vi "Deserialized data to complex.vi"(8 "error in (no error)":errorcluster, 11 "Deserialized Data In":refnum<class "3D Array s16.lvclass">) -> (0 "error out":errorcluster, 3 "Complex Data Out":refnum<class "2D Array c32.lvclass">)   [LabVIEW 2020, in "GPU FFT Calculator.lvlib" / "GPU FFT Calculator.lvclass"]
uses:
  GPU FFT Calculator.lvclass
  <vilib>/Natan Biesmans/G2CPU GPU and CPU HPC Toolkit/G2CPU Libraries/Arrays/2DArray/c32/2D Array c32.lvclass
  C:/Program Files/National Instruments/LabVIEW 2026/vi.lib/Natan Biesmans/G2CPU GPU and CPU HPC Toolkit/G2CPU Libraries/Arrays/Array/Array Prototype.lvclass
  <vilib>/Natan Biesmans/G2CPU GPU and CPU HPC Toolkit/G2CPU Libraries/Arrays/3DArray/s16/3D Array s16.lvclass
  <vilib>/Natan Biesmans/G2CPU GPU and CPU HPC Toolkit/G2CPU Libraries/Arrays/Array/Array Prototype.lvclass/Array Prototype.ctl
  c2dea994-931f-4d55-9a20-c830c6c0dc8e.vi
  b42d50d8-b553-4447-b6c3-f1e712b09a3a.vi
  a356b423-7bdc-4f21-90e1-9c0ca5a82237.vi
  d3968e77-9a7a-4b56-abf9-f7dead729653.vi
  <vilib>/Natan Biesmans/G2CPU GPU and CPU HPC Toolkit/G2CPU Libraries/Arrays/Array/G2CPU Get Array Pointer.vi
  c2dea994-931f-4d55-9a20-c830c6c0dc8e.vi/e7247370-a01f-465a-ac0e-4dfefcb1bb87.vi
  c2dea994-931f-4d55-9a20-c830c6c0dc8e.vi/345e91f0-9a5e-4de4-af9c-133346717e4a.vi
  b42d50d8-b553-4447-b6c3-f1e712b09a3a.vi/2e03f477-51b7-4ba0-bb4f-4f838f6557e6.vi
  b42d50d8-b553-4447-b6c3-f1e712b09a3a.vi/0be70a8c-200c-453e-b8ff-fd186066a0ad.vi
  b42d50d8-b553-4447-b6c3-f1e712b09a3a.vi/e82a863a-43d4-4d21-a8d3-9b1c3ad7b341.vi
  b42d50d8-b553-4447-b6c3-f1e712b09a3a.vi/99530adb-fade-452a-867c-88e355f5b47e.vi
  <vilib>/Natan Biesmans/G2CPU GPU and CPU HPC Toolkit/ArrayFire Driver/VIs/release array.vi
  b42d50d8-b553-4447-b6c3-f1e712b09a3a.vi/9eb95f43-766d-4b65-bcfe-7bdf0b763efe.vi
  b42d50d8-b553-4447-b6c3-f1e712b09a3a.vi/125d45d4-836b-469d-8a4a-6adb452f866d.vi
  b42d50d8-b553-4447-b6c3-f1e712b09a3a.vi/8038e9ed-2e71-4568-91ba-0d873494c5ed.vi
  a356b423-7bdc-4f21-90e1-9c0ca5a82237.vi/2e03f477-51b7-4ba0-bb4f-4f838f6557e6.vi
  a356b423-7bdc-4f21-90e1-9c0ca5a82237.vi/0be70a8c-200c-453e-b8ff-fd186066a0ad.vi
  a356b423-7bdc-4f21-90e1-9c0ca5a82237.vi/e82a863a-43d4-4d21-a8d3-9b1c3ad7b341.vi
  a356b423-7bdc-4f21-90e1-9c0ca5a82237.vi/99530adb-fade-452a-867c-88e355f5b47e.vi
  a356b423-7bdc-4f21-90e1-9c0ca5a82237.vi/9eb95f43-766d-4b65-bcfe-7bdf0b763efe.vi
  a356b423-7bdc-4f21-90e1-9c0ca5a82237.vi/125d45d4-836b-469d-8a4a-6adb452f866d.vi
  a356b423-7bdc-4f21-90e1-9c0ca5a82237.vi/8038e9ed-2e71-4568-91ba-0d873494c5ed.vi
  d3968e77-9a7a-4b56-abf9-f7dead729653.vi/03bcaf7a-f997-40c7-aa5f-ee6794298837.vi
  d3968e77-9a7a-4b56-abf9-f7dead729653.vi/ce8d10de-c2d8-4b5f-bf63-496f7ec21db6.vi
  d3968e77-9a7a-4b56-abf9-f7dead729653.vi/fb64f27e-acf2-4ea7-8121-5cd3b475beac.vi
  d3968e77-9a7a-4b56-abf9-f7dead729653.vi/79c68e2d-670c-4431-8d6a-9dd6c37feee1.vi
  b42d50d8-b553-4447-b6c3-f1e712b09a3a.vi/2e03f477-51b7-4ba0-bb4f-4f838f6557e6.vi/d8e2d9cc-c923-495e-b121-b6b84788c73f.vi
  b42d50d8-b553-4447-b6c3-f1e712b09a3a.vi/2e03f477-51b7-4ba0-bb4f-4f838f6557e6.vi/345e91f0-9a5e-4de4-af9c-133346717e4a.vi
  <vilib>/Natan Biesmans/G2CPU GPU and CPU HPC Toolkit/ArrayFire Driver/VIs/Run as Multi Device.vi
  <vilib>/Natan Biesmans/G2CPU GPU and CPU HPC Toolkit/G2CPU Libraries/Runtime Licensing/G2CPU License Check.vi
  b42d50d8-b553-4447-b6c3-f1e712b09a3a.vi/125d45d4-836b-469d-8a4a-6adb452f866d.vi/1b7cf390-2ae0-48f3-9bce-03c57eed6ee8.vi
  a356b423-7bdc-4f21-90e1-9c0ca5a82237.vi/2e03f477-51b7-4ba0-bb4f-4f838f6557e6.vi/d8e2d9cc-c923-495e-b121-b6b84788c73f.vi
  a356b423-7bdc-4f21-90e1-9c0ca5a82237.vi/2e03f477-51b7-4ba0-bb4f-4f838f6557e6.vi/345e91f0-9a5e-4de4-af9c-133346717e4a.vi
  a356b423-7bdc-4f21-90e1-9c0ca5a82237.vi/125d45d4-836b-469d-8a4a-6adb452f866d.vi/1b7cf390-2ae0-48f3-9bce-03c57eed6ee8.vi
  d3968e77-9a7a-4b56-abf9-f7dead729653.vi/79c68e2d-670c-4431-8d6a-9dd6c37feee1.vi/3e802c67-fb96-46a3-ae13-4994a8508b4f.vi
  d3968e77-9a7a-4b56-abf9-f7dead729653.vi/79c68e2d-670c-4431-8d6a-9dd6c37feee1.vi/5a50fc67-79e7-4972-80c2-92243cd53dd4.vi
  <vilib>/Natan Biesmans/G2CPU GPU and CPU HPC Toolkit/G2CPU Libraries/Arrays/3DArray/f32/3D Array f32.lvclass
  <vilib>/Natan Biesmans/G2CPU GPU and CPU HPC Toolkit/G2CPU Libraries/Arrays/1DArray/u32/1D Array u32.lvclass
  <vilib>/Natan Biesmans/G2CPU GPU and CPU HPC Toolkit/G2CPU Libraries/Arrays/1DArray/s32/1D Array s32.lvclass
  <vilib>/Natan Biesmans/G2CPU GPU and CPU HPC Toolkit/G2CPU Libraries/Arrays/2DArray/f32/2D Array f32.lvclass
  <vilib>/Natan Biesmans/G2CPU GPU and CPU HPC Toolkit/ArrayFire Driver/VIs/cast.vi
  <vilib>/Natan Biesmans/G2CPU GPU and CPU HPC Toolkit/G2CPU Libraries/Arrays/Array/G2CPU Set Array Pointer.vi
  <vilib>/Natan Biesmans/G2CPU GPU and CPU HPC Toolkit/ArrayFire Driver/subvi/Error Converter (ErrCode or Status).vi
  <vilib>/Natan Biesmans/G2CPU GPU and CPU HPC Toolkit/ArrayFire Driver/VIs/lookup.vi
  <vilib>/Natan Biesmans/G2CPU GPU and CPU HPC Toolkit/G2CPU Libraries/Arrays/SubVI/RemoveReducedDimensionForReorder.vi
  <vilib>/Natan Biesmans/G2CPU GPU and CPU HPC Toolkit/ArrayFire Driver/VIs/reorder.vi
  <vilib>/Natan Biesmans/G2CPU GPU and CPU HPC Toolkit/G2CPU Libraries/Arrays/SubVI/G2CPU State.vi
  <vilib>/NI License Manager/Open Session.vi
  <vilib>/NI License Manager/Check License Status.vi
  <vilib>/NI License Manager/Check License Status (Single).vi
  <vilib>/NI License Manager/Activate License.vi
  <vilib>/NI License Manager/Activate License (Single).vi
  <vilib>/NI License Manager/Close Session.vi
  <vilib>/Natan Biesmans/G2CPU GPU and CPU HPC Toolkit/ArrayFire Driver/VIs/cplx2.vi
  <vilib>/Natan Biesmans/G2CPU GPU and CPU HPC Toolkit/G2CPU Libraries/Arrays/Array/Array Prototype.lvclass
  <vilib>/Natan Biesmans/G2CPU GPU and CPU HPC Toolkit/G2CPU Libraries/Arrays/3DArray/3D Array Prototype.lvclass
  <vilib>/Natan Biesmans/G2CPU GPU and CPU HPC Toolkit/G2CPU Libraries/Arrays/DataTypes/I32/s32.lvclass
  <vilib>/Natan Biesmans/G2CPU GPU and CPU HPC Toolkit/G2CPU Libraries/Arrays/1DArray/1D Array Prototype.lvclass
  <vilib>/Natan Biesmans/G2CPU GPU and CPU HPC Toolkit/G2CPU Libraries/Arrays/DataTypes/f32/f32.lvclass
  <vilib>/Natan Biesmans/G2CPU GPU and CPU HPC Toolkit/G2CPU Libraries/Arrays/2DArray/2D Array Prototype.lvclass
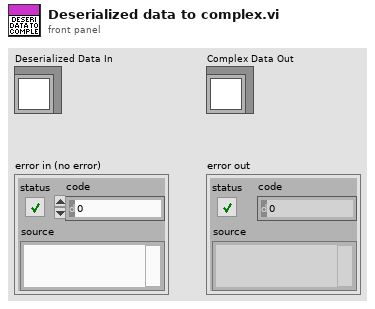
[diagram p1: front panel]
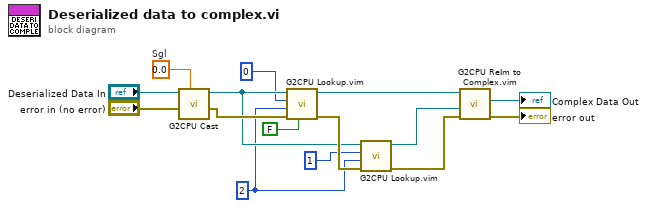
[diagram p0: block diagram]
diagram:
  w5 = u64 2 ("dim")
  w1 = sgl 0.0  # Sgl
  n1 = call "G2CPU Cast"("Datatype Prototype"=w1, "error in (no error)"="error in (no error)", "Array In"="Deserialized Data In") -> ("error out"=w7:errorcluster, "Array Out"=w6:refnum<class "3D Array f32.lvclass">)  [unwired: 7 in]
  n2 = call "G2CPU Lookup.vim"("Auto Release Array In (Enabled)"=FALSE, "error in (no error)"=w7, "dim"=w5, "Indices (1D)"=u32 0, "Array In"=w6) -> ("error out"=w8:errorcluster, "Indexed Array"=w13:refnum<class "2D Array f32.lvclass">)  [unwired: 5 in]
  n3 = call "G2CPU Lookup.vim"("error in (no error)"=w8, "dim"=w5, "Indices (1D)"=u32 1, "Array In"=w6) -> ("error out"=w15:errorcluster, "Indexed Array"=w14:refnum<class "2D Array f32.lvclass">)  [unwired: 6 in]
  n4 = call "G2CPU ReIm to Complex.vim"("error in (no error)"=w15, "Array Imaginary"=w14, "Array Real"=w13) -> ("error out"=→"error out":errorcluster, "Array Result"=→"Complex Data Out":refnum<class "2D Array c32.lvclass">)  [unwired: 7 in]
